vi "test_array_constant.vi"   [LabVIEW 2012]
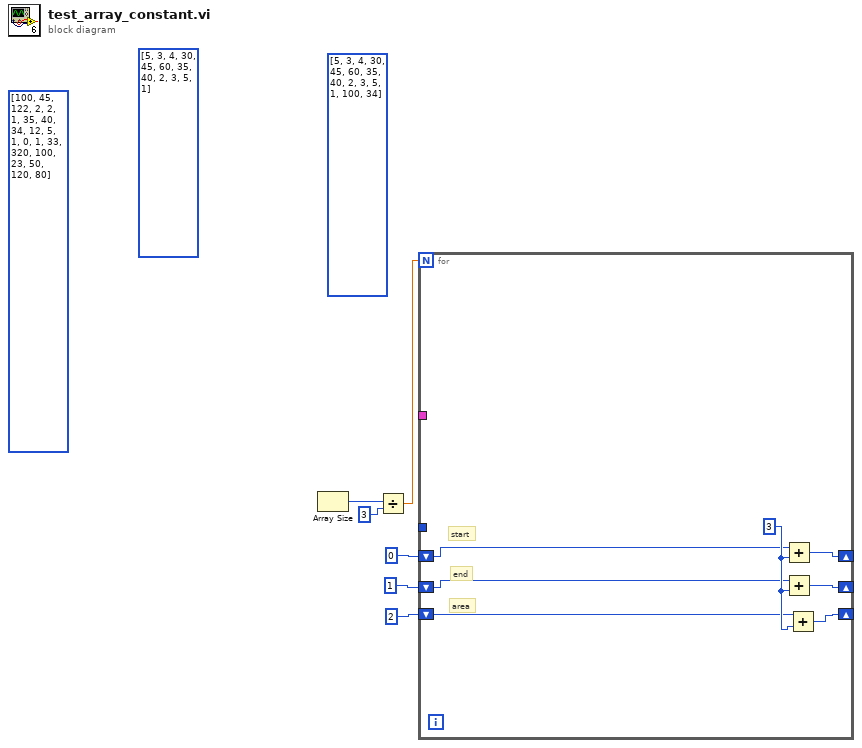
[diagram p0: block diagram]
diagram:
  (unwired) i16[] [100, 45, 122, 2, 2, 1, 35, 40, 34, 12, 5, 1, 0, 1, 33, 320, 100, 23, 50, 120, 80]
  w9 = i16[] [5, 3, 4, 30, 45, 60, 35, 40, 2, 3, 5, 1, 100, 34]
  w10 = i16[] [5, 3, 4, 30, 45, 60, 35, 40, 2, 3, 5, 1]
  n1 = Array Size() -> (size(s)=w8:i32)  [unwired: 1 in]
  n2 = Divide(x=w8, y=3) -> (x/y=w1:dbl)
  n3 = for {
    N: w1 -> [_]
    tunnel: [_] -> w2
    shift-right: [w13] -> _
    shift-left: 0 ("y") -> [w16]
    shift-right: [w12] -> _
    shift-left: 1 ("y") -> [w15]
    shift-right: [w11] -> _
    shift-left: 2 ("y") -> [w14]
    tunnel: [_] -> w3
    w17 = 3 ("y")
    # "area"
    # "end"
    # "start"
    n4 = Add(x=w16, y=w17) -> (x+y=w13:i32)
    n5 = Add(x=w15, y=w17) -> (x+y=w12:i32)
    n6 = Add(x=w14, y=w17) -> (x+y=w11:i32)
  }
